vi "AOS.vi"(0 "System no.":i32=1 min=1 max=4 step=1, 2 "Axes to set":string[](array[string]), 3 "Analog offset values":dbl[](array[numeric]) format="%.6f", 4 "No.of digits":i16=4, 5 "error in":errorcluster) -> (19 "error out":errorcluster)   [LabVIEW 2020]
doc: "Set Analog Input Offset. This command adds an offset value to an input value of an analog input, which is configured as analog target position for the selected axis. The target position of the selected axis is Target = Analog Input + Offset. No. of digits is the number of digits after the decimal point in the position value(s) that will be sent."
panel:
  # "Sets analog input offset."
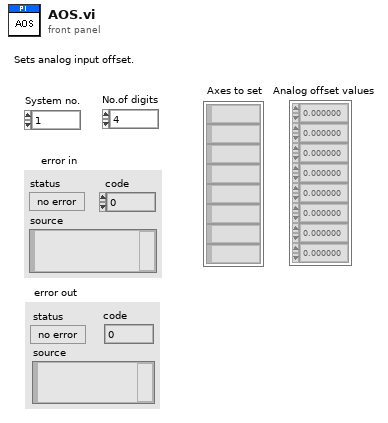
[diagram p1: front panel]
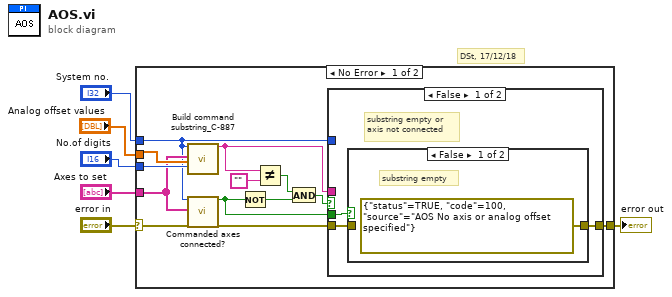
[diagram p0: block diagram]
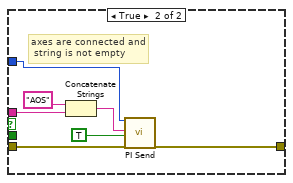
[diagram p3: hidden frame]
diagram:
  # "DSt, 17/12/18"
  n1 = case shown="No Error" "error in" {
    selector: "error in" -> [w7 w32]
    tunnel: [w19 w32] -> w6
    tunnel: "Analog offset values" -> [w16 _]
    tunnel: "No.of digits" -> [w15 _]
    tunnel: "System no." -> [w8 _]
    tunnel: "Axes to set" -> [w13 _]
    frame No Error {
      n2 = call "Build command substring_C-887.vi"("System no."=w8, "Affected axes"=w13, "Parameters"=w16, "No. of digits"=w15) -> ("Command substring"=w17:string)  [unwired: 3 in, 12 out]
      n3 = call "Commanded axes connected?.vi"("System no."=w8, "Commanded axes"=w13, "error in"=w7) -> ("Controller error"=w11:bool, "error out"=w14:errorcluster)  [unwired: 1 in, 14 out]
      n4 = Not(x=w11) -> (.not. x?=w10:bool)
      n5 = Not Equal?(x=w17, y="") -> (x != y?=w12:bool)
      n6 = And(x=w12, y=w10) -> (x .and. y?=w9:bool)
      n7 = case shown="False" w9 {
        tunnel: w17 -> [_ w30]
        tunnel: [w22 w26] -> w19
        tunnel: w14 -> [w20 w27]
        tunnel: w11 -> [w21 _]
        tunnel: w8 -> [_ w25]
        frame False {
          # "substring empty or \naxis not connected"
          n8 = case shown="False" w21 {
            tunnel: [errorcluster {"status"=TRUE, "code"=100, "source"="AOS No axis or analog offset specified"} ("error out") w24] -> w22
            tunnel: w20 -> [_ w24]
            frame False {
              # "substring empty"
            }
            frame True {
              # "commanded axis\nnot connected"
            }
          }
        }
        frame True {
          # "axes are connected and\n string is not empty"
          n9 = Concatenate Strings("AOS", w30) -> (w28:string)
          n10 = call "PI Send.vi"("System no."=w25, "String to send"=w28, "Attach termination char.?"=TRUE ("Attach Linefeed?"), "error in"=w27) -> ("error out"=w26:errorcluster)  [unwired: 2 in, 13 out]
        }
      }
    }
    frame Error {
    }
  }
  "error out" <- w6
